vi "ReadIVBuffers.vi"(8 "error in (no error)":errorcluster, 10 "XYGraph Refnum":refnum<vi>, 11 "VISA Refnum in":refnum<visa-resource-name>) -> (0 "error out":errorcluster, 3 "Array":dbl[][](array[numeric]))   [LabVIEW 2020]
uses:
  Keithley 2600 Series/Keithley 2600 Series.lvlib
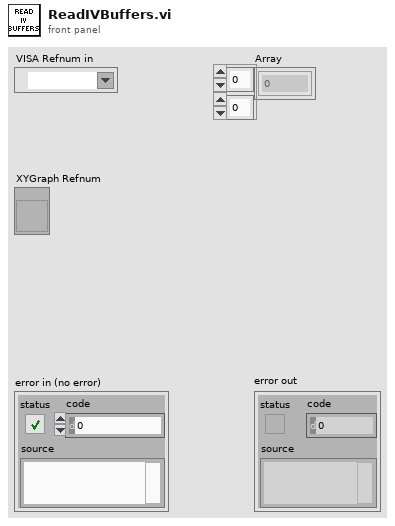
[diagram p1: front panel]
types:
  T1 = cluster{"array type (2D Dbl)":dbl[], "array type (2D Dbl)":dbl[]}
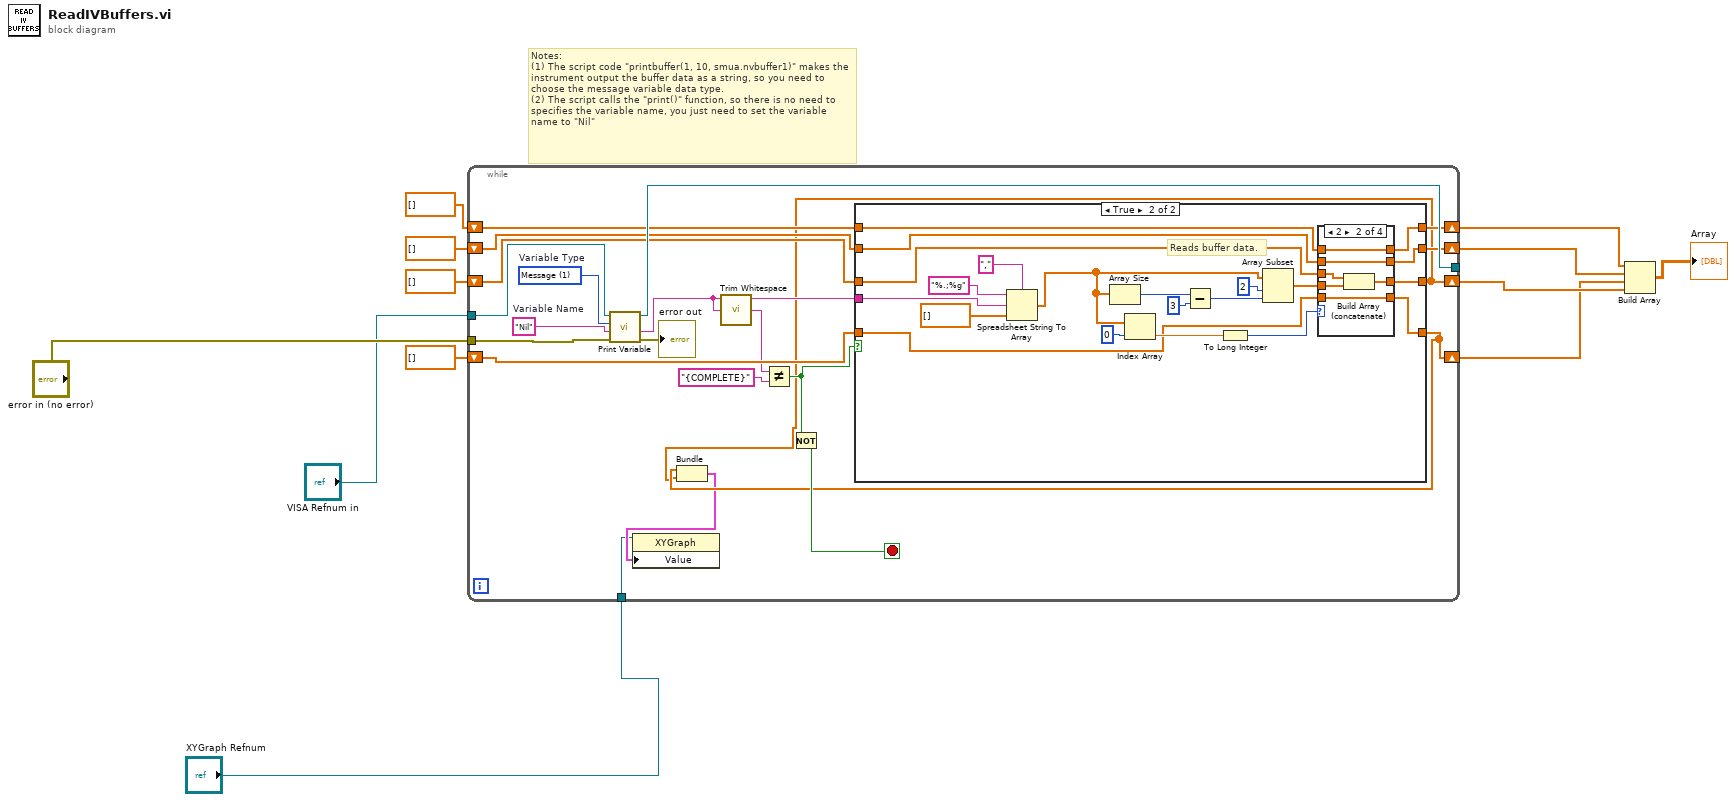
[diagram p0: block diagram]
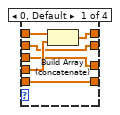
[diagram p3: hidden frame]
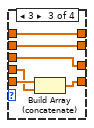
[diagram p4: hidden frame]
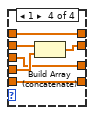
[diagram p5: hidden frame]
diagram:
  # "Notes: \n(1) The script code \"printbuffer(1, 10, smua.nvbuffer1)\" makes the instrument output the buffer data as a string, so you need to choose the message variable data type.\n(2) The script calls the \"print()\" function, so there is no need to specifies the variable name, you just need to set the variable name to \"Nil\""
  n1 = while {
    tunnel: "VISA Refnum in" -> [w31]
    tunnel: [w29] -> _
    shift-right: [w24] -> w7
    shift-left: dbl[] [] ("array type (2D Dbl)") -> [w25]
    shift-right: [w16] -> w9
    shift-left: dbl[] [] ("array type (2D Dbl)") -> [w23]
    shift-right: [w28] -> w6
    shift-left: dbl[] [] ("array type (2D Dbl)") -> [w27]
    shift-right: [w15] -> w10
    shift-left: dbl[] [] ("array type (2D Dbl)") -> [w26]
    tunnel: "error in (no error)" -> [w17]
    tunnel: "XYGraph Refnum" -> [w13]
    stop <- w18 stop-if-true
    w33 = 1 items=["Number", "Message"]  # Variable Type
    w32 = "Nil"  # Variable Name
    n2 = call "Print Variable.vi"("error in (no error)"=w17, "Variable Name"=w32, "Variable Type (0: Number)"=w33, "VISA resource name"=w31) -> ("error out"=→"error out":errorcluster, "Message"=w22:string, "VISA resource name out"=w29:refnum<visa-resource-name>)  [unwired: 4 in, 1 out]
    n3 = call <vilib>:"Trim Whitespace.vi"("string"=w22) -> ("trimmed string"=w21:string)  [unwired: 1 in]
    n4 = Not Equal?(x=w21, y="{COMPLETE}") -> (x != y?=w19:bool)
    n5 = Not(x=w19) -> (.not. x?=w18:bool)
    n6 = case shown="True" w19 {
      tunnel: w22 -> [_ w55]
      tunnel: [w37 w53] -> w28
      tunnel: w27 -> [w37 w52]
      tunnel: [w35 w50] -> w15
      tunnel: w26 -> [w35 w48]
      tunnel: w25 -> [w36 w47]
      tunnel: [w36 w46] -> w24
      tunnel: w23 -> [w34 w45]
      tunnel: [w34 w44] -> w16
      frame False {
      }
      frame True {
        # "Reads buffer data."
        n7 = Spreadsheet String To Array(delimiter (Tab)=",", format string="%.;%g", spreadsheet string=w55, array type (2D Dbl)=dbl[] []) -> (array=w41:dbl[])
        n8 = Array Size(array=w41) -> (size(s)=w40:i32)
        n9 = Index Array(array=w41, index=0) -> (element=w51:dbl)
        n10 = Subtract(x=w40, y=3) -> (x-y=w38:i32)
        n11 = To Long Integer(number=w51) -> (32bit integer=w49:i32)
        n12 = Array Subset(array=w41, index=2, length=w38) -> (w43:dbl[])
        n13 = case shown="2" w49 {
          tunnel: [w62 w70 w76 w82] -> w53
          tunnel: w52 -> [w64 w70 w76 w82]
          tunnel: [w61 w65 w75 w78] -> w50
          tunnel: w43 -> [w63 w68 w72 w80]
          tunnel: w48 -> [w61 w69 w75 w78]
          tunnel: w47 -> [w60 w67 w74 w81]
          tunnel: [w60 w67 w74 w79] -> w46
          tunnel: w45 -> [w59 w66 w73 w77]
          tunnel: [w59 w66 w71 w77] -> w44
          frame 0, Default {
            n14 = Build Array (concatenate)(w64, w63) -> (w62:dbl[])
          }
          frame 2 {
            n15 = Build Array (concatenate)(w69, w68) -> (w65:dbl[])
          }
          frame 3 {
            n16 = Build Array (concatenate)(w73, w72) -> (w71:dbl[])
          }
          frame 1 {
            n17 = Build Array (concatenate)(w81, w80) -> (w79:dbl[])
          }
        }
      }
    }
    n18 = Bundle("array type (2D Dbl)"=w16, "array type (2D Dbl)"=w15) -> (w14:T1)  [unwired: 1 in]
    n19 = property class="XYGraph"(reference=w13, "Value"=w14) -> ()  [unwired: 1 in, 2 out]
  }
  n20 = Build Array(w6, w7, w9, w10) -> (→"Array":dbl[][])
